vi "Calculation for heating 4 vessel (SILAR).vi"(0 "Tz - заданная температура":dbl, 1 "Tt - текущая температура":dbl, 2 "Ttp - текущая (прошлая) температура":dbl, 3 "Tsp - суммарная (прошлая) температура":dbl, 4 "tp - время прошлое":dbl, 5 "tn - время настоящее":dbl) -> (14 "t1 - время во включенном состоянии":dbl, 19 "Ts - суммарная температура":dbl)   [LabVIEW 2016]
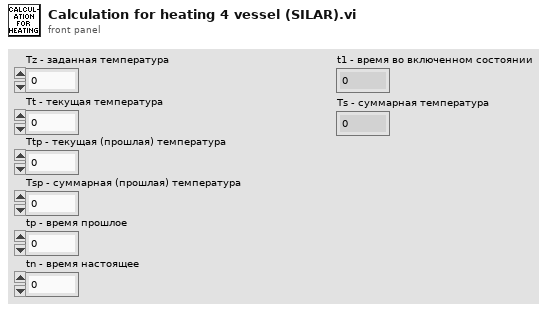
[diagram p1: front panel]
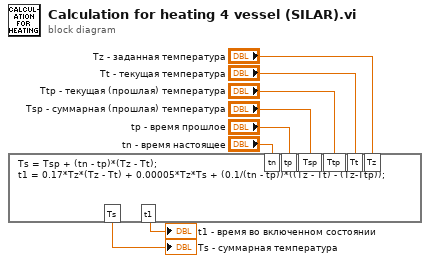
[diagram p0: block diagram]
diagram:
  n1 = formula code="Ts = Tsp + (tn - tp)*(Tz - Tt);\nt1 = 0.17*Tz*(Tz - Tt) + 0.00005*Tz*Ts + (0.1/(tn - tp))*((Tz - Tt) - (Tz-Ttp));"("Tz"="Tz - заданная температура", "Tt"="Tt - текущая температура", "Ttp"="Ttp - текущая (прошлая) температура", "Tsp"="Tsp - суммарная (прошлая) температура", "tp"="tp - время прошлое", "tn"="tn - время настоящее") -> ("t1"=→"t1 - время во включенном состоянии":dbl, "Ts"=→"Ts - суммарная температура":dbl)
